vi "Window.vi"(0 "VISA IN":refnum<visa-resource-name>, 5 "error in":errorcluster, 6 "Window\nCreate(ON)/Delete(OFF)":bool, 7 "Window":i32=1, 9 "Window Size":string(combo)="NORM", 11 "Window Arrangement":string(combo)="QUAD") -> (14 "VISA Out":refnum<visa-resource-name>, 19 "error out":errorcluster)   [LabVIEW 2018, in "PNA-X.lvlib"]
uses:
  PNA-X.lvlib
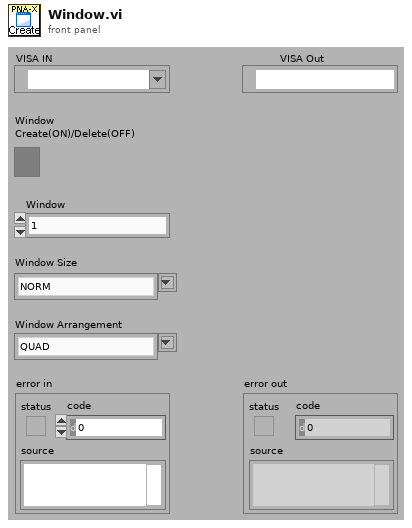
[diagram p1: front panel]
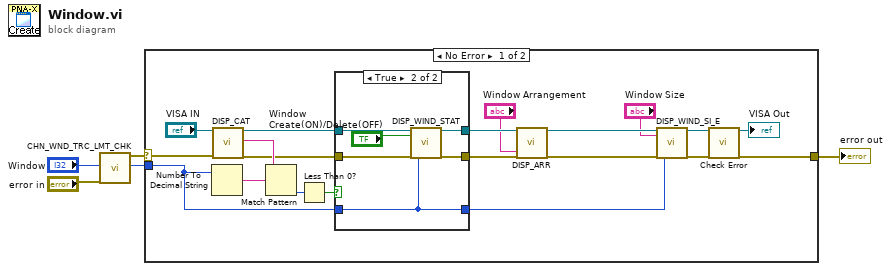
[diagram p0: block diagram]
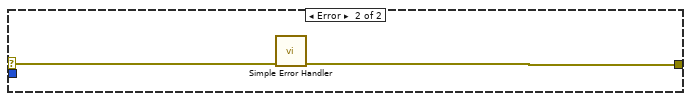
[diagram p3: hidden frame]
diagram:
  n1 = call "CHN_WND_TRC_LMT_CHK.vi"("Window"="Window", "error in"="error in") -> ("error out"=w2:errorcluster, "Window"=w1:i32)  [unwired: 13 in, 3 out]
  n2 = case shown="No Error" w2 {
    selector: w2 -> [w22 w36]
    tunnel: [w25 w35] -> w4
    tunnel: w1 -> [w15 _]
    frame No Error {
      n3 = Number To Decimal String(number=w15) -> (decimal integer string=w21:string)  [unwired: 1 in]
      n4 = call "DISP_CAT.vi"("VISA IN"="VISA IN", "error in"=w22) -> ("VISA Out"=w18:refnum<visa-resource-name>, "Data"=w19:string, "error out"=w17:errorcluster)  [unwired: 15 in]
      n5 = Match Pattern(string=w19, regular expression=w21) -> (offset past match=w20:i32)  [unwired: 1 in, 3 out]
      n6 = Less Than 0?(x=w20) -> (x < 0?=w16:bool)
      n7 = case shown="True" w16 {
        tunnel: w18 -> [w27 w33]
        tunnel: w17 -> [w28 w32]
        tunnel: [w28 w30] -> w13
        tunnel: [w27 w31] -> w14
        tunnel: w15 -> [w26 w29]
        tunnel: [w26 w29] -> w10
        frame False {
        }
        frame True {
          n8 = call "DISP_WIND_STAT.vi"("VISA IN"=w33, "ON | OFF"="Window\nCreate(ON)/Delete(OFF)", "error in"=w32, "Window"=w29) -> ("VISA Out"=w31:refnum<visa-resource-name>, "error out"=w30:errorcluster)  [unwired: 14 in]
        }
      }
      n9 = call "DISP_ARR.vi"("VISA IN"=w14, "error in"=w13, "Window Arrangement"="Window Arrangement") -> ("VISA Out"=w11:refnum<visa-resource-name>, "error out"=w12:errorcluster)  [unwired: 15 in]
      n10 = call "DISP_WIND_SI_E.vi"("VISA IN"=w11, "Size"="Window Size", "error in"=w12, "Window"=w10) -> ("VISA Out"=w8:refnum<visa-resource-name>, "error out"=w9:errorcluster)  [unwired: 14 in]
      n11 = call "Check Error.vi"("VISA Resource Name"=w8, "error in (no error)"=w9) -> ("dup VISA session"=→"VISA Out":refnum<visa-resource-name>, "error out"=w25:errorcluster)  [unwired: 16 in]
    }
    frame Error {
      n12 = call <vilib>:"Simple Error Handler.vi"("error in (no error)"=w36) -> ("error out"=w35:errorcluster)  [unwired: 4 in, 4 out]
    }
  }
  "error out" <- w4
